vi "decode_pose.vi"(11 "Ref pose":T1) -> (1 "Handle pose string":string, 2 "Translation":dbl[](array[numeric]) format="%#.1f", 3 "Handle pose":T1 format="%#.3f", 4 "Relative angles":dbl[](array[numeric]) format="%#.1f", 5 "Total angle":dbl format="%#_4g")   [LabVIEW 2013]
uses:
  <vilib>/Analysis/Matrix/Datatypes/RealMatrix.ctl
  <vilib>/Analysis/coordinate.llb/Angle Units.ctl
  <vilib>/Analysis/baseanly.llb/Real A x B.vi
  <vilib>/Analysis/coordinate.llb/Wrap Angle (array).vi
  <vilib>/Analysis/Matrix/Numeric/Conversions/Array To Matrix - RA2.vi
  <vilib>/Analysis/Matrix/NI_Matrix.lvlib
  <vilib>/Analysis/NI_AALBase.lvlib
  <vilib>/Analysis/NI_AAL_Angle.lvlib
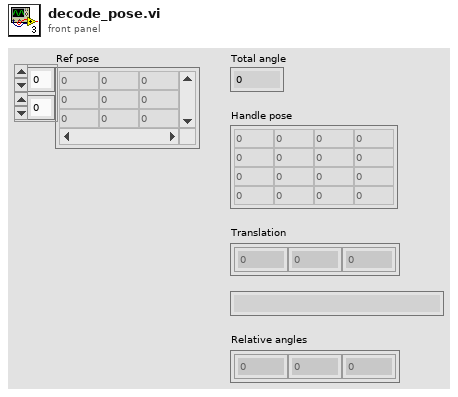
[diagram p1: front panel]
types:
  T1 = typedef "NI_Matrix.lvlib/RealMatrix.ctl" = dbl[][]
  T2 = typedef "NI_AAL_Angle.lvlib/Angle Units.ctl" = i32
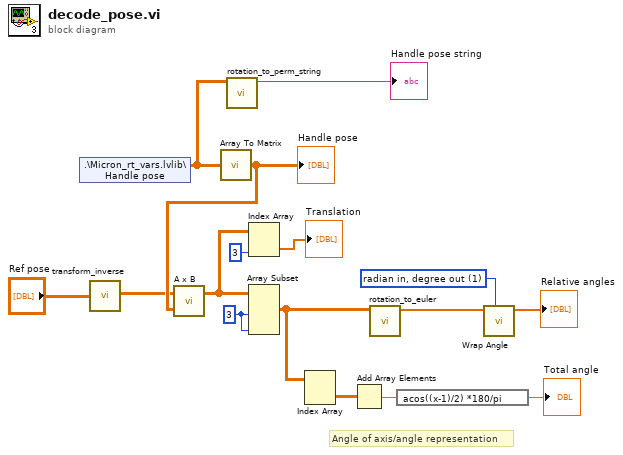
[diagram p0: block diagram]
diagram:
  w4 = T2 1 items=["radian in, radian out", "radian in, degree out", "degree in, degree out", "degree in, radian out"] ("angle units")
  w6 = 3 ("length")
  # "Angle of axis/angle representation"
  n1 = shared-variable ".\\Micron_rt_vars.lvlib\\Handle pose"() -> (w15:sgl[][])  [unwired: 1 in, 1 out]
  n2 = call "transform_inverse.vi"("Transform"="Ref pose") -> ("Inverse transform"=w2:T1)
  n3 = call-poly <vilib>:"Array To Matrix.vi"("Real 2D Array"=w15) -> ("Real Matrix"=w3:T1)
  "Handle pose" <- w3
  n4 = call-poly <vilib>:"A x B.vi"("B"=w3, "A"=w2) -> ("A x B"=w12:T1)  [unwired: 1 out]
  n5 = call "rotation_to_perm_string.vi"("Rotation matrix (T)"=w15) -> ("Axis permutation and residue"=→"Handle pose string":string)  [unwired: 10 in]
  n6 = Index Array(array=w12, index (col)=3 ("disabled index (col)")) -> (element=→"Translation":dbl[])  [unwired: 1 in]
  n7 = Array Subset(array=w12, length (row)=w6, length (col)=w6) -> (w8:T1)  [unwired: 2 in]
  n8 = Index Array(array=w8) -> (element=w9:T1)  [unwired: 2 in]
  n9 = Add Array Elements(numeric array=w9) -> (sum=w10:dbl)
  n10 = call "rotation_to_euler.vi"("Rotation"=w8) -> ("Theta XYZ"=w5:dbl[])  [unwired: 10 in]
  n11 = expression code="acos((x-1)/2) *180/pi"(w10) -> (→"Total angle":dbl)
  n12 = call-poly <vilib>:"Wrap Angle.vi"("angle units"=w4, "Angle In"=w5) -> ("Angle Out"=→"Relative angles":dbl[])  [unwired: 8 in, 1 out]
